vi "General Globals.vi"() -> ()   [LabVIEW 2017]
uses:
  Peripherals Control/Shutter/Typedefs/Shutter state.ctl
  Typedefs/Top level VI states.ctl
panel:
  in  "Axial Scanning":bool
  in  "Initial Laser wavelength":i32=900
  in  "Initial dwell time [us]":dbl=0.1
  in  "Initial Acceptance Angle":i32=5
  in  "Initial Scan Resolution":i32=512
  in  "Advanced Imaging":bool
  out "Microscope Type":string
  out "Microscope ID":string
  in  "User Folder Path":path
  in  "Software Revision Number":string
  in  "Delete accidental time series":bool
  in  "Generate user folder?":bool
  in  "Daily folder path":path
  in  "Filename of loaded user profile":string
  out "Funct.acq. TDMS refs":refnum<k34>[](array[refnum])
  out "Acq Module's State":string
  in  "Close":bool
  out "Protocol status":string
  in  "Chirps on Restart":bool
  in  "Restart":bool
  in  "Ref plots window bring to front":bool
  in  "Ref plots window is open":bool
  in  "Ref plots window-Open":bool
  in  "Show ref plots window":bool
  in  "DevPC - No hardware":bool
  in  "Func.acq. ref frame save is enabled":bool=TRUE
  in  "Last State":T1
  out "Stop ref imaging window":bool
  in  "Funct.acq post-proc enabled":bool=TRUE
  in  "Live window is open":bool
  in  "Timelapse frames saved":u32
  in  "Last experiment folder path":path
  in  "Close message window":bool
  in  "Video recording enabled":bool
  in  "Save MC TestData":bool
  in  "Generating Z-ztack Chirps":bool
  in  "Regenerate chirps":bool
  in  "Generating Chirps":bool
  in  "First autogen":bool
  in  "Background MovCor window is open":bool
  in  "Background MovCor":bool
  in  "AO Sample Clock Rate (samples/sec)":dbl=1000000.0 format="%#_6f"
  in  "Timelapse folder path":path
  out "# Planes":i32
  in  "Base path":path
  in  "Max allowed trial length (sec)":dbl=60.0 format="%#_13g"
  in  "Hardware limitation (number of lines across al ROI)":i32=1024
  in  "Acquisition completed":bool
  in  "Objective":string(combo)="Olympus  20X"
  in  "Config Files Folder Path":path
  out "Protocol start timestamp":timestamp
  out "Center Frequency":dbl=39.0
  in  "Virtual shutter state":T2
  in  "Live Imaging":bool
  in  "Snapshot Ref":bool
  in  "Snapshot":bool
  in  "PacketHeader":string
  in  "Movement Correction":bool
  in  "Subpanel is open":bool
  in  "Stop subpanel":bool
  in  "Timelapse?":bool
  in  "Reset to slow speed":bool
  in  "AOD fill time (us)":dbl=24.5
  in  "Timelapse path generated":bool
  in  "Timelapse count":u32
  in  "Speed logging enabled":bool
  in  "Speed graph window is open":bool
  in  "Open speed graph window":bool
  in  "Abort low priority processes":bool
  in  "Logging process is active":bool
  in  "Progress bar window is open":bool
  in  "Stop application":bool
  # "WARNING!\nDO NOT RENAME THIS GLOBAL VARIABLE VI BECAUSE A COMMON VI IN THE USER.LLB IS EXPECTING THIS NAME\n\"GENERAL GLOBALS\"."
  # "<----Temporary global\nTo be replaced by the AOL globals FG"
  # "These are settings"
  # "<-- Use the FGV instead"
  # "<-- Use the FGV instead"
  # "<-- This counts the number of frames \nin the current AVI split file."
  # "<-- Use the FGV instead"
  # "<--- Calculated. Centre frequency(MHz) = AOL wavelength(nm) * AOL centre frequency(MHz) / UI wavelength (nm)\nFor debugging purposes only. Use AOL globals instead."
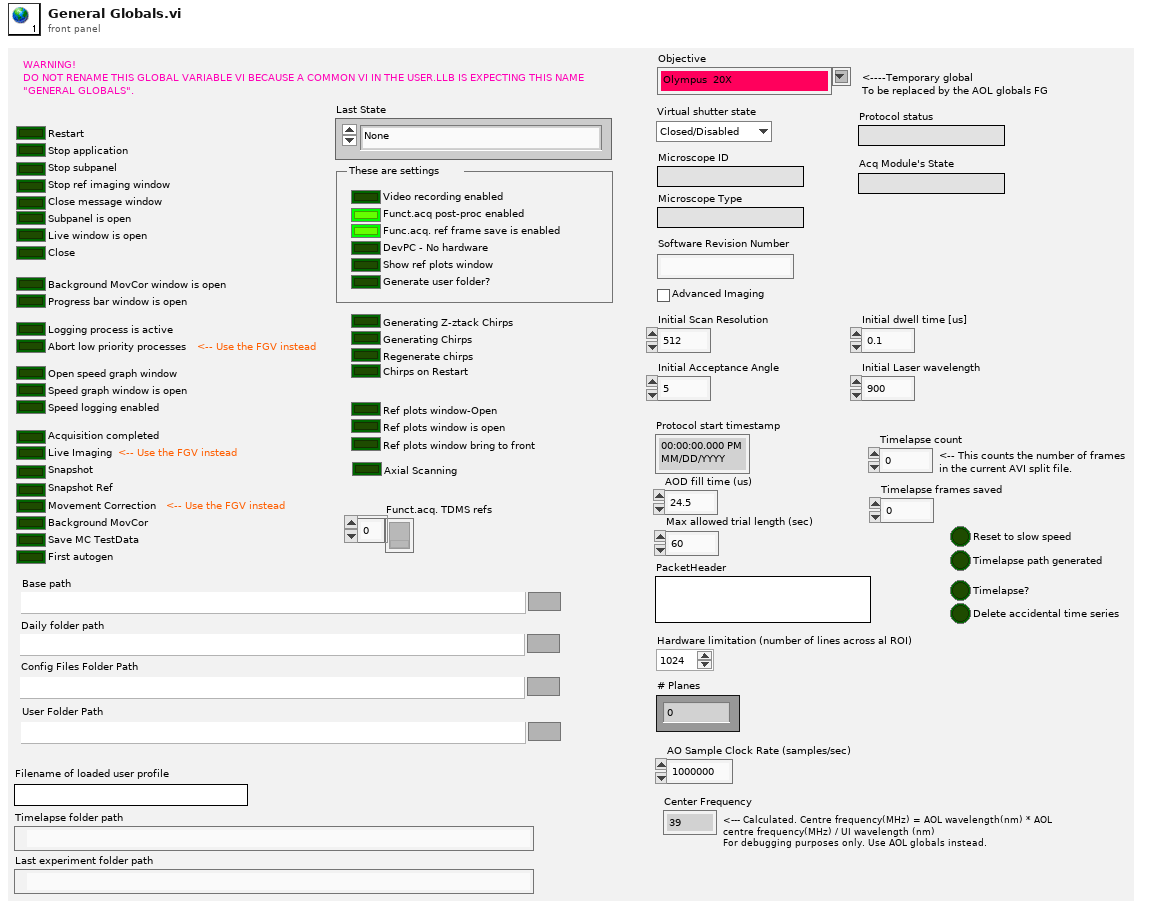
[diagram p1: front panel]
types:
  T1 = typedef "Top level VI states.ctl" = enum16{"None", "Initialise UI", "<STACK PROTOCOL STATES>", "AOL Zstack-START", "AOL Zstack-STOP", "Motor Zstack-START", "Motor Zstack-STOP", "<ACQUISITION PROTOCOL STATES> ", "Functional Acquisition-START", "Functional Acquisition-STOP", "Single Plane Acquisition-START", "Single Plane Acquisition-STOP", "Volume Acquisition-START", "Volume Acquisition-STOP", "<LIVE IMAGING PROTOCOL STATES>", "Live Imaging-START", "Live Imaging-STOP", "Live Plane Imaging-START", "Live Plane Imaging-STOP", "Live Volume Imaging-START", "Live Volume Imaging-STOP", "<MOVEMENT CORRECTION PROTOCOL STATES>", "EXIT"}
  T2 = typedef "Shutter state.ctl" = enum16{"Closed/Disabled", "Open/Enabled"}
diagram:
